vi "Read Network Master.vi"(8 "error in (no error)":errorcluster, 11 "TCP in":refnum<class "TCP.lvclass">) -> (0 "error out":errorcluster, 2 "Network Master":refnum<class "Network Master.lvclass">, 3 "TCP out":refnum<class "TCP.lvclass">)   [LabVIEW 2021, in "TCP.lvclass"]
uses:
  TCP.lvclass
  D:/my_projects/projects/Algorithms/Labview/21/Master CR/Master CR.lvclass
  Modbus_v121c/Network Protocol/Network Master/Network Master.lvclass
  Master CR.lvclass/Master CR.ctl
  TCP.lvclass/TCP.ctl
  Master CR.lvclass
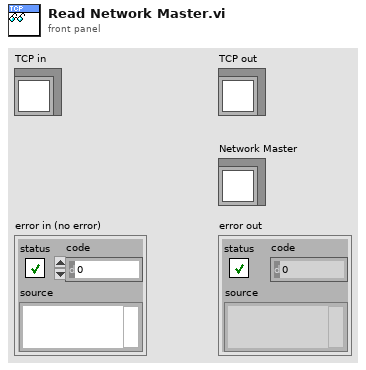
[diagram p1: front panel]
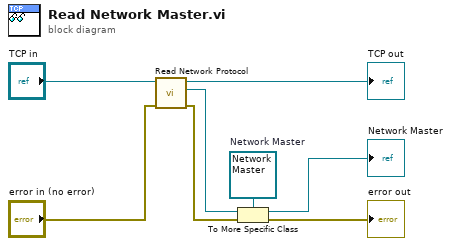
[diagram p0: block diagram]
diagram:
  w5 = refnum<class "Network Master.lvclass"> refnum  # Network Master
  n1 = call "Read Network Protocol.vi"("error in (no error)"="error in (no error)", "Master CR in"="TCP in") -> ("error out"=w3:errorcluster, "Network Protocol"=w4:refnum<class "Network Protocol.lvclass">, "Master CR out"=→"TCP out":refnum<class "TCP.lvclass">)  [unwired: 7 in]
  n2 = To More Specific Class(target class=w5, reference=w4, error in=w3) -> (specific class reference=→"Network Master":refnum<class "Network Master.lvclass">, error out=→"error out":errorcluster)
